vi "Ring Ref Update Color.vi"(8 "error in (no error)":errorcluster, 11 "Num ref":refnum<vi>) -> (0 "error out":errorcluster)   [LabVIEW 2018, in "Main Panel.lvlib" / "Main Panel.lvclass"]
uses:
  Main Panel.lvclass
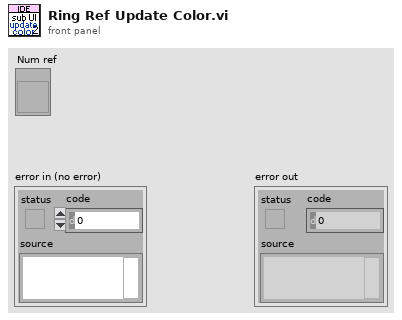
[diagram p1: front panel]
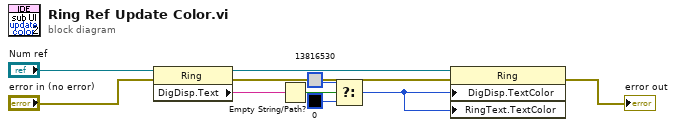
[diagram p0: block diagram]
diagram:
  n1 = property class="Ring"(reference="Num ref", error in="error in (no error)") -> (reference out=w7:refnum<vi>, error out=w3:errorcluster, "DigDisp.Text"=w2:string)
  n2 = Empty String/Path?(string/path=w2) -> (empty?=w6:bool)
  n3 = Select(t=u32 13816530, s=w6, f=u32 0) -> (s? t:f=w1:u32)
  n4 = property class="Ring"(reference=w7, error in=w3, "DigDisp.TextColor"=w1, "RingText.TextColor"=w1) -> (error out=→"error out":errorcluster)  [unwired: 1 out]
